vi "PH_Synchrolock_Watch.ProcPeriodic.vi"(0 "i ref in":refnum<vi>, 3 "ms timeout (10000)":i32=10000, 5 "error in (no error)":errorcluster) -> (14 "i ref out":refnum<vi>, 17 "timed out":bool, 19 "error out":errorcluster)   [LabVIEW 2014, in "PH_Synchrolock_Watch.lvlib"]
doc: "This method serves to periodically do things like reading values from the HW. Methods that should be executed periodically should be called from THIS methode. Add code here."
uses:
  PH_Synchrolock_Watch.lvlib
  PH_Devices/PH_TKTDS-30xx/PH_TKTDS-30xx.Channel Config.ctl
  PH_Devices/PH_TKTDS-30xx/PH_TKTDS-30xx.Waveform Limits.ctl
  PH_Devices/PH_TKTDS-30xx/PH_TKTDS-30xx.lvlib
  CS_Core/CSSystem/CSSystemLib/CSSystemLib.lvlib
panel:
  in  "Array":T3(array[cluster]) {"Channel Configuration"."Vertical Offset" format="%#_6p"; "Channel Configuration"."Vertical Range" items=["1mV"=0.001, "2mV"=0.002, "5mV"=0.005, "10mV"=0.01, "20mV"=0.02, "50mV"=0.05, "100mV"=0.1, "200mV"=0.2, "500mV"=0.5, "1V"=1.0]; "Channel Configuration"."Probe Attenuation" format="%#.2f"}
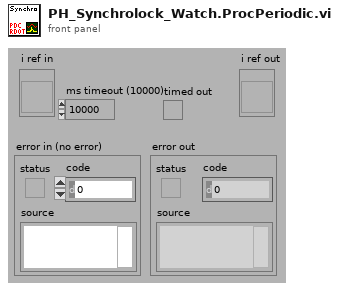
[diagram p1: front panel]
types:
  T1 = typedef "PH_TKTDS-30xx.lvlib/PH_TKTDS-30xx.Channel Config.ctl" = cluster{"Channel Name":string, "Input Impedance":string, "Max Input Frequency":string, "Vertical Coupling":i32, "Channel Enabled":bool, "Probe Attenuation":dbl, "Vertical Range":dbl, "Vertical Offset":dbl, "Waveform Limits":T2}
  T2 = typedef "PH_TKTDS-30xx.lvlib/PH_TKTDS-30xx.Waveform Limits.ctl" = cluster{"Start":i32, "End":i32}
  T3 = cluster{"High Energy GUI Element Name":string, "Channel Configuration":T1}[]
  T4 = typedef "PH_TKTDS-30xx.lvlib/PH_TKTDS-30xx.i attribute.ctl" = cluster{"Default VISA Resource":string, "VISA Resource Name":refnum<visa-resource-name>, "Revision":cluster{"Instrument Driver":string, "Instrument Firmware":string}, "Selftest":cluster{"Result":u32, "Message":string}, "Channels":T1[], "Trigger Configuration":T5, "Acquisition Configuration":T6, "Fetched Waveforms":T7[], "GUI Refs":T8, "State":T9, "Error Message":string, "Allow Prdc Loop?":bool}
  T5 = typedef "PH_TKTDS-30xx.lvlib/PH_TKTDS-30xx.Trigger Config.ctl" = cluster{"Source":string, "Slope":i32, "Level [V]":dbl}
  T6 = typedef "PH_TKTDS-30xx.lvlib/PH_TKTDS-30xx.Acquisition Config.ctl" = cluster{"Time base":dbl, "Record Length":u16, "Start Time":dbl, "Type":i32, "Continuous":bool}
  T7 = typedef "PH_TKTDS-30xx.lvlib/PH_TKTDS-30xx.fetched Waveform.ctl" = cluster{"Source":string, "Actual Points":u32, "Initial X":dbl, "X Increment":dbl, "Waveform Array":dbl[]}
  T8 = typedef "PH_TKTDS-30xx.lvlib/PH_TKTDS-30xx.GUI Refs.ctl" = cluster{"Trigger":refnum<vi>, "Acquisition":refnum<vi>, "State":refnum<vi>, "Delete":refnum<vi>, "Channel to be positioned":refnum<vi>, "Postion":refnum<vi>, "Display Intensity":refnum<vi>, "VISA Resource":refnum<vi>, "Channels":refnum<vi>[], "Graphs":refnum<vi>[]}
  T9 = typedef "PH_StatusHandler.lvlib/PH_StatusHandler.Status.ctl" = i16
  T10 = cluster{"Label.Text":string, "Channel Configuration":T1}
  T11 = cluster{"Label.Text":string, "Channel Configuration":T1}[]
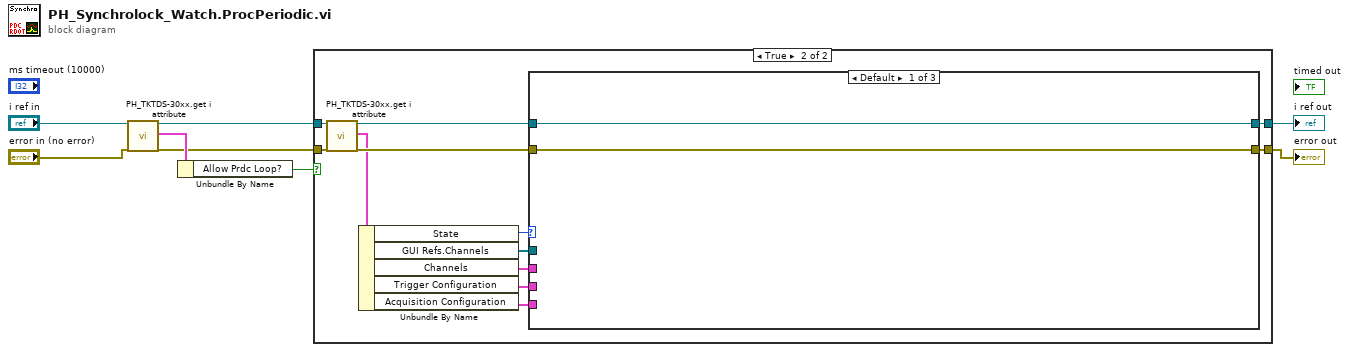
[diagram p0: block diagram]
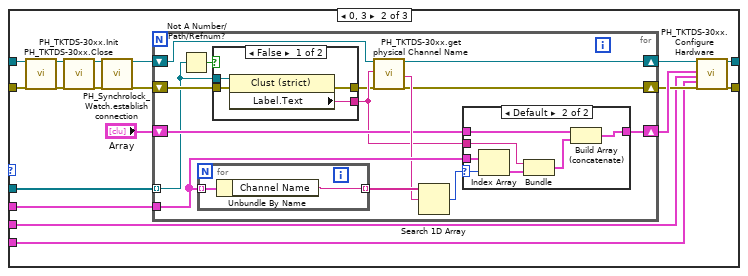
[diagram p3: hidden frame]
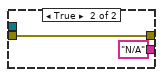
[diagram p4: hidden frame]
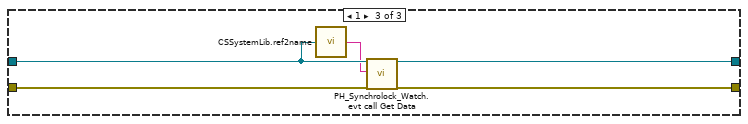
[diagram p6: hidden frame]
diagram:
  n1 = call "PH_TKTDS-30xx.get i attribute.vi"("i ref in"="i ref in", "error in (no error)"="error in (no error)") -> ("i ref out"=w3:refnum<vi>, "i attribute"=w6:T4, "error out"=w4:errorcluster)  [unwired: 15 in]
  n2 = Unbundle By Name(w6) -> ("Allow Prdc Loop?"=w5:bool)
  n3 = case shown="True" w5 {
    tunnel: w3 -> [w10 w21]
    tunnel: [w10 w20] -> w1
    tunnel: [w9 w18] -> w2
    tunnel: w4 -> [w9 w17]
    frame False {
    }
    frame True {
      n4 = call "PH_TKTDS-30xx.get i attribute.vi"("i ref in"=w21, "error in (no error)"=w17) -> ("i ref out"=w22:refnum<vi>, "i attribute"=w16:T4, "error out"=w19:errorcluster)  [unwired: 15 in]
      n5 = Unbundle By Name(w16) -> ("State"=w15:T9, "GUI Refs.Channels"=w14:refnum<vi>[], "Channels"=w13:T1[], "Trigger Configuration"=w12:T5, "Acquisition Configuration"=w11:T6)
      n6 = case shown="Default" w15 {
        tunnel: w22 -> [w24 w38 w74]
        tunnel: [w24 w36 w76] -> w20
        tunnel: w19 -> [w23 w41 w77]
        tunnel: [w23 w35 w75] -> w18
        tunnel: w14 -> [_ w30 _]
        tunnel: w13 -> [_ w29 _]
        tunnel: w12 -> [_ w28 _]
        tunnel: w11 -> [_ w27 _]
        frame Default {
        }
        frame 0, 3 {
          n7 = call "PH_TKTDS-30xx.Close.vi"("i ref in"=w38, "error in(no error)"=w41) -> ("i ref out"=w37:refnum<vi>, "error out"=w39:errorcluster)  [unwired: 16 in]
          n8 = call "PH_TKTDS-30xx.Init.vi"("i ref in"=w37, "error in (no error)"=w39) -> ("i ref out"=w42:refnum<vi>, "error out"=w40:errorcluster)  [unwired: 16 in]
          n9 = call "PH_Synchrolock_Watch.establish connection.vi"("i ref in"=w42, "error in"=w40) -> ("i ref out"=w26:refnum<vi>, "error out"=w25:errorcluster)  [unwired: 16 in]
          n10 = for {
            tunnel: w29 -> [w55]
            shift-right: [w53] -> w33
            shift-left: w26 -> [w43]
            shift-right: [w52] -> w32
            shift-left: w25 -> [w46]
            shift-right: [w51] -> w34
            shift-left: "Array" -> [w50]
            tunnel: w30 -> [w44] mode=indexing
            n11 = Not A Number/Path/Refnum?(number/path/refnum=w44) -> (NaN/Path/Refnum?=w48:bool)
            n12 = for {
              tunnel: w55 -> [w72] mode=indexing
              tunnel: [w71] -> w56 mode=indexing
              n13 = Unbundle By Name(w72) -> ("Channel Name"=w71:string)
            }
            n14 = case shown="False" w48 {
              tunnel: w46 -> [w60 w62]
              tunnel: [w59 w62] -> w45
              tunnel: [w58 "N/A" ("Label.Text")] -> w47
              tunnel: w44 -> [w57 _]
              frame False {
                n15 = property class="Clust (strict)"(reference=w57, error in=w60) -> (error out=w59:errorcluster, "Label.Text"=w58:string)  [unwired: 1 out]
              }
              frame True {
              }
            }
            n16 = call "PH_TKTDS-30xx.get physical Channel Name.vi"("i ref in"=w43, "GUI Element Name"=w47, "error in"=w45) -> ("i ref out"=w53:refnum<vi>, "Physical Channel Name"=w54:string, "error out"=w52:errorcluster)  [unwired: 13 in, 1 out]
            n17 = Search 1D Array(1D array=w56, element=w54) -> (index of element=w49:i32)  [unwired: 1 in]
            n18 = case shown="Default" w49 {
              selector: w49 -> [_ w64]
              tunnel: w55 -> [_ w70]
              tunnel: w47 -> [_ w67]
              tunnel: [w63 w66] -> w51
              tunnel: w50 -> [w63 w65]
              frame -1 {
              }
              frame Default {
                n19 = Index Array(array=w70, index=w64) -> (element=w69:T1)
                n20 = Bundle("Label.Text"=w67, "Channel Configuration"=w69) -> (w68:T10)  [unwired: 1 in]
                n21 = Build Array (concatenate)(w65, w68) -> (w66:T11)
              }
            }
          }
          n22 = call "PH_TKTDS-30xx.Configure Hardware.vi"("i ref in"=w33, "Channels Sets"=w34, "Trigger Settings"=w28, "Acqu Settings"=w27, "error in"=w32) -> ("i ref out"=w36:refnum<vi>, "error out"=w35:errorcluster)  [unwired: 13 in]
        }
        frame 1 {
          n23 = call "CSSystemLib.ref2name.vi"("obj refnum"=w74) -> ("name"=w73:string)
          n24 = call "PH_Synchrolock_Watch.evt call Get Data.vi"("i ref in"=w74, "Instance"=w73, "error in (no error)"=w77) -> ("i ref out"=w76:refnum<vi>, "error out"=w75:errorcluster)  [unwired: 15 in]
        }
      }
    }
  }
  "error out" <- w2
  "i ref out" <- w1
